vi "Create NI-XNET Session.vi"(8 "Error In":errorcluster, 11 "NI-XNET Port In":refnum<k21>) -> (0 "Error Out":errorcluster, 3 "Session out":refnum<k21>)   [LabVIEW 2018, in "NI-XNET Monitor Engine.lvlib"]
uses:
  NI-XNET Monitor Engine.lvlib
  <vilib>/xnet/xnet.llb/XNET Create Session (Frame Input Stream).vi
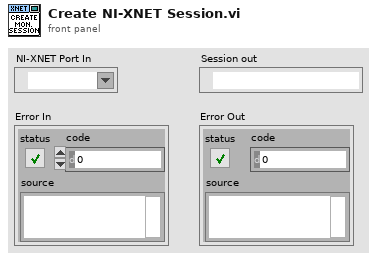
[diagram p1: front panel]
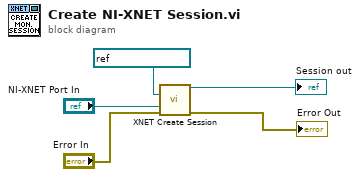
[diagram p0: block diagram]
diagram:
  n1 = call-poly <vilib>:"XNET Create Session.vi"("cluster (:memory:)"=refnum<k21> ":subordinate:" ("cluster out"), "interface"="NI-XNET Port In", "error in (no error)"="Error In") -> ("session out"=→"Session out":refnum<k21>, "error out"=→"Error Out":errorcluster)  [unwired: 11 in]
